vi "手动启动选择对话框.vi"() -> (2 "确定":bool, 3 "参数":T2)   [LabVIEW 2016, in "PLC.lvlib"]
uses:
  PLC.lvlib
panel:
  in  "自动运行启动参数":T1
  in  "测试模式":enum16{"正常测试", "集成干预"}(ring)
  in  "取消":bool
  in  "确定":bool
  # "请选择启动参数"
  # "请选择启动模式："
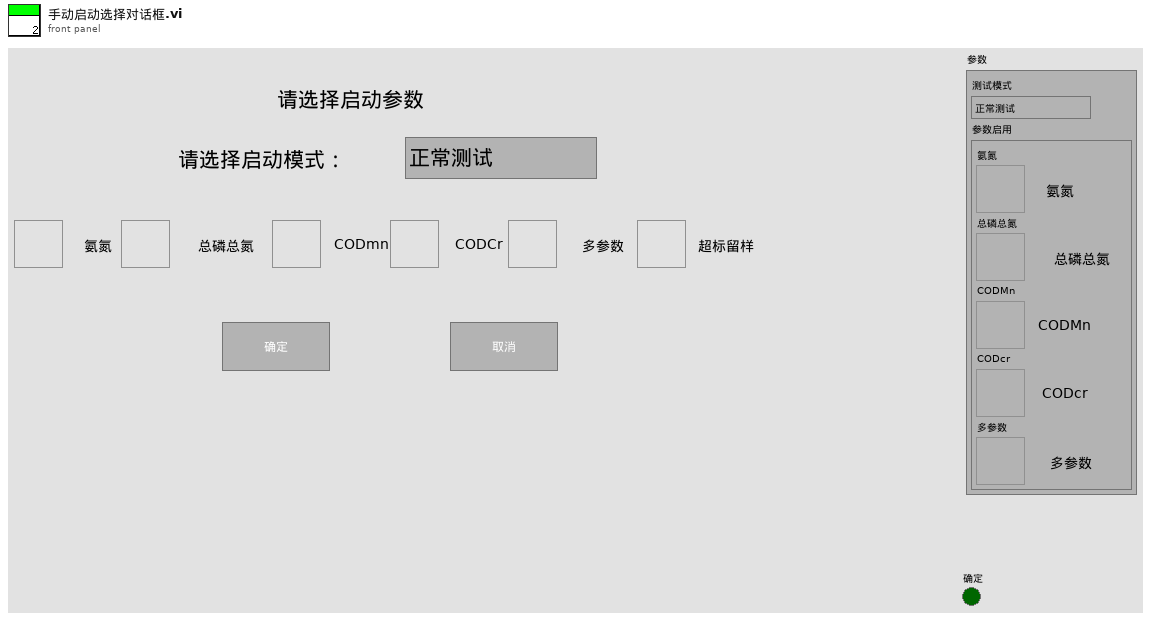
[diagram p1: front panel]
types:
  T1 = cluster{"氨氮":bool, "总磷总氮":bool, "CODmn":bool, "CODCr":bool, "多参数":bool, "超标留样":bool}
  T2 = cluster{"测试模式":enum16{"正常测试", "集成干预"}, "参数启用":cluster{"氨氮":bool, "总磷总氮":bool, "CODMn":bool, "CODcr":bool, "多参数":bool, "超标留样":bool}}
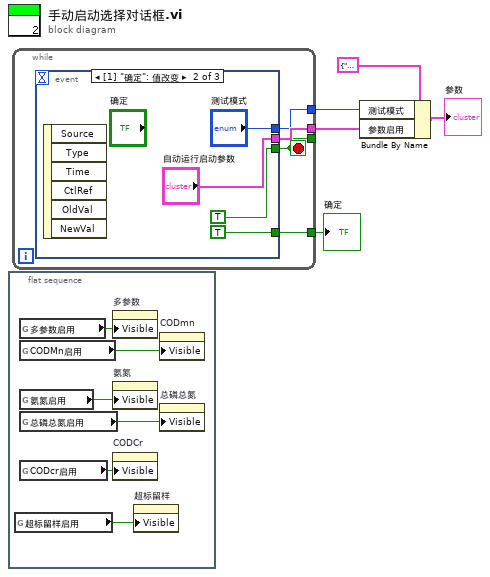
[diagram p0: block diagram]
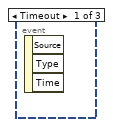
[diagram p2: hidden frame]
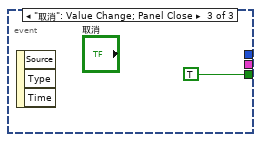
[diagram p3: hidden frame]
diagram:
  n1 = flat-sequence {
    frame #0 {
      n2 = global read "系统设置全局变量.vi" "超标留样启用"() -> (w6:bool)
      n3 = global read "系统设置全局变量.vi" "多参数启用"() -> (w8:bool)
      n4 = global read "系统设置全局变量.vi" "CODMn启用"() -> (w10:bool)
      n5 = global read "系统设置全局变量.vi" "氨氮启用"() -> (w9:bool)
      n6 = global read "系统设置全局变量.vi" "总磷总氮启用"() -> (w7:bool)
      n7 = global read "系统设置全局变量.vi" "CODcr启用"() -> (w11:bool)
      n8 = property on="多参数" class="Bool (严格)"("Visible"=w8) -> ()  [unwired: 2 in, 2 out]
      n9 = property on="氨氮" class="Bool (严格)"("Visible"=w9) -> ()  [unwired: 2 in, 2 out]
      n10 = property on="CODCr" class="Bool (严格)"("Visible"=w11) -> ()  [unwired: 2 in, 2 out]
      n11 = property on="超标留样" class="Bool (严格)"("Visible"=w6) -> ()  [unwired: 2 in, 2 out]
      n12 = property on="CODmn" class="Bool (严格)"("Visible"=w10) -> ()  [unwired: 2 in, 2 out]
      n13 = property on="总磷总氮" class="Bool (严格)"("Visible"=w7) -> ()  [unwired: 2 in, 2 out]
    }
  }
  n14 = while {
    tunnel: [w15] -> w3
    tunnel: [w14] -> _
    tunnel: [w13] -> w5
    tunnel: [w12] -> w4
    stop <- w14 stop-if-true
    n15 = event shown="[1] \"确定\": 值改变" {
      selector: _ -> [_ _ _]
      dyn-events: _ -> [_ _ _]
      timeout: _ -> [_ _ _]
      tunnel: [_ TRUE TRUE] -> w14
      tunnel: [_ "自动运行启动参数" _] -> w15
      tunnel: [_ TRUE _] -> w13
      tunnel: [_ "测试模式" _] -> w12
      event Timeout {
        n16 = event-data() -> ()  [unwired: 1 in, 3 out]
      }
      event "确定": Value Change {
        n17 = event-data() -> ()  [unwired: 1 in, 6 out]
      }
      event "取消": Value Change; Panel Close {
        n18 = event-data() -> ()  [unwired: 1 in, 3 out]
      }
    }
  }
  "确定" <- w5
  n19 = Bundle By Name(cluster=T2 {"测试模式"=enum."正常测试", "参数启用"={"氨氮"=FALSE, "总磷总氮"=FALSE, "CODMn"=FALSE, "CODcr"=FALSE, "多参数"=FALSE, "超标留样"=FALSE}} ("参数"), "测试模式"=w4, "参数启用"=w3) -> (→"参数":T2)
